vi "Send Rotation Data.vi"(10 "DVR In":refnum<data-value>) -> ()   [LabVIEW 2016]
uses:
  Rotation Notifier.ctl
  Rotation Control Type.ctl
  Rotation Globals.vi
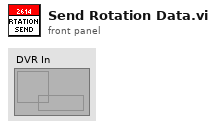
[diagram p1: front panel]
types:
  T1 = typedef "Rotation Notifier.ctl" = cluster{"Up":bool, "Down":bool, "Rotation Control List":T2, "Control Down":bool, "Manual":bool}
  T2 = typedef "Rotation Control Type.ctl" = enum16{"No Op", "Up", "Down", "Control Up", "Control Down"}
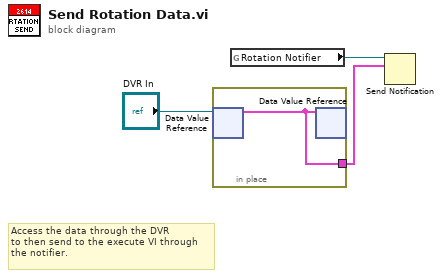
[diagram p0: block diagram]
diagram:
  # "Access the data through the DVR\nto then send to the execute VI through\nthe notifier."
  n1 = in-place {
    in-place-border: [w4] -> w3
    n2 = in-place-dvr #1("DVR In") -> (w4:T1)  [unwired: 1 out]
    n3 = in-place-dvr #1(w4) -> ()  [unwired: 2 out]
  }
  n4 = global read "Rotation Globals.vi" "Rotation Notifier"() -> (w1:refnum<notifier>)
  n5 = Send Notification(notification=w3, notifier=w1) -> ()  [unwired: 1 in, 2 out]
